vi "Digilent Basic IO Shield - OLED Draw Bool Array.vi"(8 "Error In":errorcluster, 10 "Image Data":bool[][](array[boolean]), 11 "LINX Resource":T1) -> (0 "Error Out":errorcluster, 3 "LINX Resource":T1)   [LabVIEW 2014, in "LMH-LINX.lvlib" / "SSD1306.lvlib"]
uses:
  <vilib>/MakerHub/LINX/Public/Sensors/Display/SSD1306/SSD1306.lvlib
  <vilib>/MakerHub/LINX/Private/Type Defs/Platform.ctl
  <vilib>/MakerHub/LINX/LMH-LINX.lvlib
  <vilib>/MakerHub/LINX/Private/Type Defs/Interface.ctl
  <vilib>/MakerHub/LINX/Private/Device/Type Defs/TCP Config.ctl
  <vilib>/MakerHub/LINX/Private/Device/Device.lvlib
  <vilib>/MakerHub/LINX/Private/Device/Type Defs/LINX Device Config.ctl
  <vilib>/MakerHub/LINX/Private/Type Defs/LINX Ref.ctl
  <vilib>/MakerHub/LINX/Private/Device/Type Defs/Channels.ctl
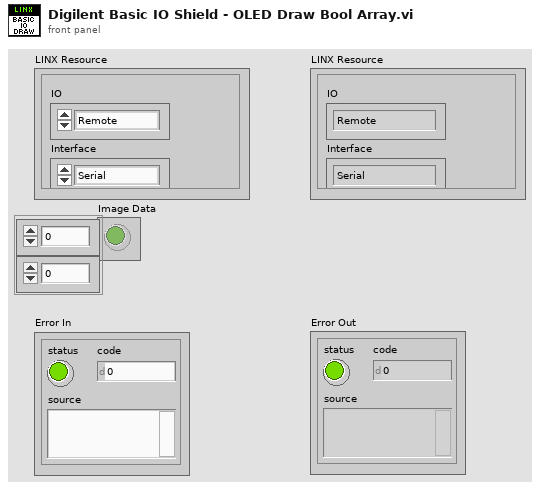
[diagram p1: front panel]
types:
  T1 = typedef "LMH-LINX.lvlib/LINX Ref.ctl" = cluster{"IO":T2, "Interface":T3, "LINX Device Config":T4}
  T2 = typedef "LMH-LINX.lvlib/Platform.ctl" = enum16{"Remote", "Local"}
  T3 = typedef "LMH-LINX.lvlib/Interface.ctl" = enum16{"Serial", "TCP"}
  T4 = typedef "LMH-LINX.lvlib/Device.lvlib/LINX Device Config.ctl" = cluster{"Interface":T3, "COM Port":refnum<visa-resource-name>, "TCP Configuration":T5, "Device Family":u8, "Device ID":u8, "Device Name":string, "TCP Ref":refnum<k5>, "Channels":T6}
  T5 = typedef "LMH-LINX.lvlib/Device.lvlib/TCP Config.ctl" = cluster{"IP Address":string, "Port":u16}
  T6 = typedef "LMH-LINX.lvlib/Channels.ctl" = cluster{"DI":u8[], "DO":u8[], "AI":u8[], "AO":u8[], "PWM":u8[], "QE":u8[], "UART":u8[], "I2C 2":u8[], "SPI":u8[], "CAN":u8[], "Servo":u8[], "AI Ref (V)":dbl, "AO Ref (V)":dbl, "AO Resolution (Bits)":u8}
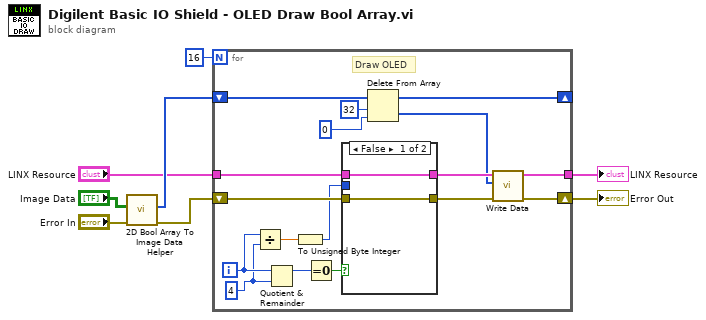
[diagram p0: block diagram]
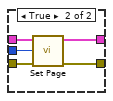
[diagram p2: hidden frame]
diagram:
  n1 = call <vilib>:"2D Bool Array To Image Data Helper.vi"("Error In"="Error In", "Image Data"="Image Data") -> ("Error Out"=w5:errorcluster, "Image Data"=w4:u8[])  [unwired: 8 in]
  n2 = for {
    N: 16 -> [_]
    tunnel: "LINX Resource" -> [w18]
    shift-right: [w14] -> _
    shift-left: w4 -> [w15]
    shift-right: [w10] -> w7
    shift-left: w5 -> [w23]
    tunnel: [w9] -> w6
    i -> [w22]
    w21 = 4 ("y")
    # "Draw OLED"
    n3 = Divide(x=w22, y=w21) -> (x/y=w20:dbl)
    n4 = Quotient & Remainder(x=w22, y=w21) -> (x-y*floor(x/y)=w25:i32)  [unwired: 1 out]
    n5 = To Unsigned Byte Integer(number=w20) -> (unsigned 8bit integer=w19:u8)
    n6 = Equal To 0?(x=w25) -> (x = 0?=w24:bool)
    n7 = case shown="False" w24 {
      tunnel: w23 -> [w26 w32]
      tunnel: w19 -> [_ w31]
      tunnel: w18 -> [w27 w30]
      tunnel: [w26 w29] -> w17
      tunnel: [w27 w28] -> w16
      frame False {
      }
      frame True {
        n8 = call <vilib>:"Set Page.vi"("Error In"=w32, "Page Address"=w31, "LINX Resource"=w30) -> ("Error Out"=w29:errorcluster, "LINX Resource"=w28:T1)  [unwired: 7 in]
      }
    }
    n9 = Delete From Array(array=w15, length=32, index=0) -> (deleted portion=w11:u8[], array with subset deleted=w14:u8[])
    n10 = call <vilib>:"Write Data.vi"("Error In"=w17, "Data"=w11, "LINX Resource"=w16) -> ("Error Out"=w10:errorcluster, "LINX Resource"=w9:T1)  [unwired: 7 in]
  }
  "LINX Resource" <- w6
  "Error Out" <- w7
